vi "Read Power FIFO.vi"(8 "error in (no error)":errorcluster, 9 "Timeout (ms)":i32=100, 10 "Data in":T1[](array[typedef])=[{"measurement"=[], "dT"=0.0, "Timestamp"=0, "Read Lock"=FALSE}, {"measurement"=[], "dT"=0.0, "Timestamp"=0, "Read Lock"=FALSE}], 11 "CIFTag in":refnum<class "CIF_NIChn_Fifo_Power.lvclass">) -> (0 "error out":errorcluster, 1 "timed out?":bool, 2 "Data out":T1[](array[typedef]), 3 "CIFTag out":refnum<class "CIF_NIChn_Fifo_Power.lvclass">, 4 "Header":T2)   [LabVIEW 2021, in "CIF_NIChn_Fifo_Power.lvclass"]
uses:
  CIF_NIChn_Fifo_Power.lvclass
  D:/dev/Packages/Channel_Manager/src/CIFChannels/CIFChannels.lvclass
  D:/dev/Packages/Channel_Manager/src/CIF_NIChn/NIChn/CIF_NIChn.lvclass
  ChannelCommon/typedef/FIFO Header.ctl
  ChannelCommon/typedef/Datatype Waveform.ctl
  CIFChannels/CIFChannels.lvclass/CIFChannels.ctl
  CIFChannels/Typedef/Channel State.ctl
  CIFChannels/Typedef/Direction.ctl
  NIChn/CIF_NIChn.lvclass/CIF_NIChn.ctl
  CIF_NIChn_Fifo_Power.lvclass/CIF_NIChn_Fifo_Power.ctl
  CIFChannels/Accessors/Read Channel State.vi
  CIFChannels/Accessors/Read Direction.vi
  CIFChannels/Accessors/Write Channel State.vi
  CIFChannels/Accessors/Read Tag Disconnect Behavior.vi
  <vilib>/CIF Foundation/CIF Channels/CIFChannels/Top Level/Read U8 Array.vi/4bc1c15b-36ab-481f-b8dd-c64075ce723a.vi
  <vilib>/CIF Foundation/CIF Channels/CIFChannels/Top Level/Read U8 Array.vi/d83cb72b-7713-41fc-a3d1-682de79cf574.vi
  <vilib>/CIF Foundation/CIF Channels/CIFChannels/SubVIs/Get dll Path.vi
  <vilib>/CIF Foundation/CIF Channels/CIFChannels/SubVIs/Get Requested Size.vi
  ChannelCommon/CIFFIFO/Flatten/Waveform Unflatten.vi
  CIFChannels/Accessors/Write FIFO Header.vi
  CIFChannels/Accessors/Write FIFO Timeout.vi
  ChannelCommon/Utilities/Unflatten Header.vi
  <vilib>/CIF Foundation/CIF Utilities/DataTypes/Unflatten I64.vi
  <vilib>/CIF Foundation/CIF Utilities/DataTypes/Unflatten U64.vi
  ChannelCommon/Utilities/Add Error.vi
  <vilib>/CIF Foundation/CIF Utilities/Errors/Append Error Location.vi
  NIChn/CIF_NIChn.lvclass
  CIFChannels/CIFChannels.lvclass
  <vilib>/CIF Foundation/CIF Channels/CIFChannels/CIFChannelCore.lvlib
  ChannelCommon/ChannelCommon.lvlib
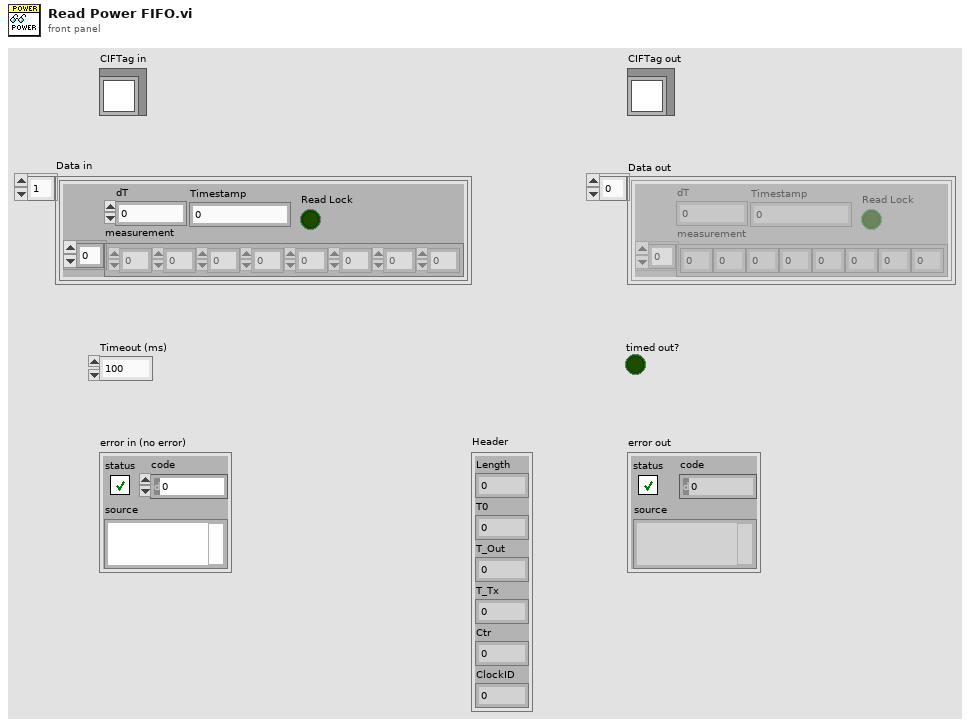
[diagram p1: front panel]
types:
  T1 = typedef "ChannelCommon.lvlib/Datatype Waveform.ctl" = cluster{"measurement":dbl[], "dT":dbl, "Timestamp":i64, "Read Lock":bool}
  T2 = typedef "ChannelCommon.lvlib/FIFO Header.ctl" = cluster{"Length":u64, "T0":i64, "T_Out":i64, "T_Tx":i64, "Ctr":u64, "ClockID":u8}
  T3 = typedef "CIFChannels.lvclass/Channel State.ctl" = enum16{"Creating", "Disconnected", "Connecting", "Connected", "Destroyed"}
  T4 = typedef "CIFChannels.lvclass/Direction.ctl" = enum16{"Publisher", "Subscriber"}
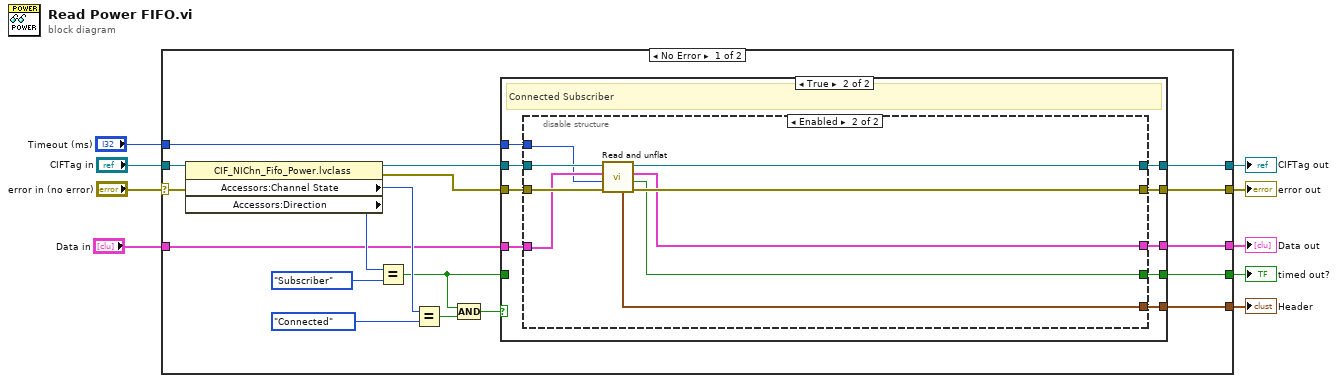
[diagram p0: block diagram]
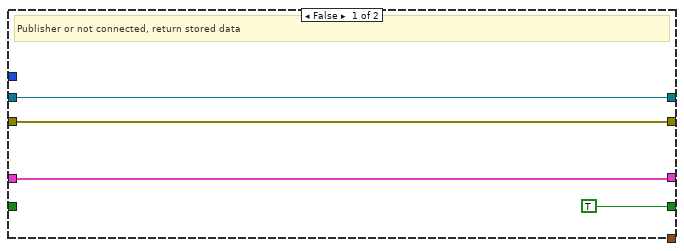
[diagram p2: hidden frame]
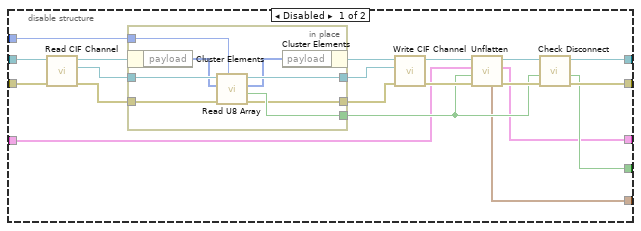
[diagram p3: hidden frame]
diagram:
  n1 = case shown="No Error" "error in (no error)" {
    selector: "error in (no error)" -> [w24 w80]
    tunnel: [w13 w80] -> w8
    tunnel: [w14 w79] -> w6
    tunnel: "CIFTag in" -> [w25 w79]
    tunnel: [w27 _] -> w5
    tunnel: [w26 w78] -> w2
    tunnel: "Timeout (ms)" -> [w12 _]
    tunnel: [w11 _] -> w3
    tunnel: "Data in" -> [w10 w78]
    frame No Error {
      n2 = property class="CIF_NIChn_Fifo_Power.lvclass"(reference=w25, error in=w24) -> (reference out=w23:refnum<class "CIF_NIChn_Fifo_Power.lvclass">, error out=w22:errorcluster, "Accessors:Channel State"=w19:T3, "Accessors:Direction"=w21:T4)
      n3 = Equal?(x=w21, y=Direction."Subscriber") -> (x = y?=w15:bool)
      n4 = Equal?(x=w19, y=Channel_State."Connected") -> (x = y?=w17:bool)
      n5 = Compound Arithmetic op=AND(w15, w17) -> (w16:bool)
      n6 = case shown="True" w16 {
        tunnel: [TRUE ("timeout out") w36] -> w27
        tunnel: [w28 w34] -> w26
        tunnel: w22 -> [w30 w39]
        tunnel: w23 -> [w31 w40]
        tunnel: w15 -> [_ _]
        tunnel: [w31 w38] -> w14
        tunnel: [w30 w37] -> w13
        tunnel: w12 -> [_ w35]
        tunnel: [_ w33] -> w11
        tunnel: w10 -> [w28 w32]
        frame False {
          # "Publisher or not connected, return stored data"
        }
        frame True {
          # "Connected Subscriber"
          n7 = disable-structure shown="Enabled" {
            disable-tunnel: w40 -> [w60 w77]
            disable-tunnel: w39 -> [w59 w76]
            disable-tunnel: [w58 w75] -> w38
            disable-tunnel: [w57 w74] -> w37
            disable-tunnel: [w50 w70] -> w36
            disable-tunnel: w35 -> [w49 w69]
            disable-tunnel: [w43 w72] -> w34
            disable-tunnel: [w42 w71] -> w33
            disable-tunnel: w32 -> [w41 w73]
            frame Disabled {
              n8 = call "Read CIF Channel.vi"("error in (no error)"=w59, "CIFTag in"=w60) -> ("error out"=w54:errorcluster, "CIF Channel"=w55:refnum<k21>, "CIFTag out"=w56:refnum<class "CIF_NIChn_Fifo_Power.lvclass">)  [unwired: 7 in]
              n9 = in-place {
                in-place-border: [w66] -> w44
                in-place-border: w55 -> [w68]
                in-place-border: w54 -> [w67]
                in-place-border: [w65] -> w51
                in-place-border: [w64] -> w52
                in-place-border: w49 -> [w63]
                n10 = in-place-cluster #1(w56) -> ("payload"=w62:u8[])
                n11 = call <vilib>:"Read U8 Array.vi"("Timeout (ms)"=w63, "error in"=w67, "U8 Array in"=w62, "CIF Channel in"=w68) -> ("error out"=w64:errorcluster, "Timed out?"=w66:bool, "U8 Array out"=w61:u8[], "CIF Channel out"=w65:refnum<k21>)  [unwired: 4 in]
                n12 = in-place-cluster #1("payload"=w61) -> (w53:refnum<class "CIF_NIChn_Fifo_Power.lvclass">)
              }
              n13 = call "Write CIF Channel.vi"("error in (no error)"=w52, "CIF Channel"=w51, "CIFTag in"=w53) -> ("error out"=w47:errorcluster, "CIFTag out"=w48:refnum<class "CIF_NIChn_Fifo_Power.lvclass">)  [unwired: 7 in]
              n14 = call "Unflatten.vi"("error in (no error)"=w47, "timeout in"=w44, "Data in"=w41, "CIFFifoCAN in"=w48) -> ("error out"=w45:errorcluster, "Data out"=w43:T1[], "CIFFifoCAN out"=w46:refnum<class "CIF_NIChn_Fifo_Power.lvclass">, "Header"=w42:T2)  [unwired: 4 in]
              n15 = call "Check Disconnect.vi"("error in (no error)"=w45, "timeout in"=w44, "CIFTag in"=w46) -> ("error out"=w57:errorcluster, "timeout out"=w50:bool, "CIFTag out"=w58:refnum<class "CIF_NIChn_Fifo_Power.lvclass">)  [unwired: 5 in, 1 out]
            }
            frame Enabled {
              n16 = call "Read and unflat.vi"("error in (no error)"=w76, "Timeout (ms)"=w69, "Data in in"=w73, "CIF_NIChn_Fifo_Power in"=w77) -> ("error out"=w74:errorcluster, "Timed out?"=w70:bool, "Data out"=w72:T1[], "CIF_NIChn_Fifo_Power out"=w75:refnum<class "CIF_NIChn_Fifo_Power.lvclass">, "Header out"=w71:T2)  [unwired: 3 in]
            }
          }
        }
      }
    }
    frame Error {
    }
  }
  "error out" <- w8
  "CIFTag out" <- w6
  "timed out?" <- w5
  "Header" <- w3
  "Data out" <- w2
